vi "To bytes if not empty.vi"(3 "MessagePack.lvlib:IMsgPackContainer.lvclass":refnum<class "IMsgPackContainer.lvclass">) -> (1 "Array":u8[](array[numeric]))   [LabVIEW 2020, in "MessagePack.lvlib"]
uses:
  MessagePack.lvlib
  IMsgPackContainer/IMsgPackContainer.lvclass
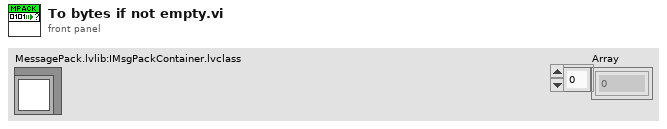
[diagram p1: front panel]
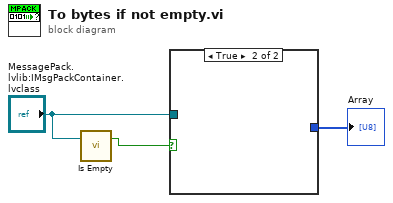
[diagram p0: block diagram]
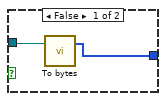
[diagram p2: hidden frame]
diagram:
  n1 = call-dynamic "Is Empty.vi"("IMsgPackContainer in"="MessagePack.lvlib:IMsgPackContainer.lvclass") -> ("Is empty?"=w3:bool)  [unwired: 2 in]
  n2 = case shown="True" w3 {
    tunnel: "MessagePack.lvlib:IMsgPackContainer.lvclass" -> [w5 _]
    tunnel: [w4 _] -> w1
    frame False {
      n3 = call-dynamic "To bytes.vi"("IMessagePackObject in"=w5) -> ("Array"=w4:u8[])  [unwired: 2 in]
    }
    frame True {
    }
  }
  "Array" <- w1
